vi "Callback.vi"(8 "error in (no error)":errorcluster, 9 "Message Data":variant, 10 "Message":string, 11 "Callback in":refnum<class "Callback.lvclass">) -> (0 "error out":errorcluster)   [LabVIEW 2020, in "Callback.lvclass"]
uses:
  Callback.lvclass
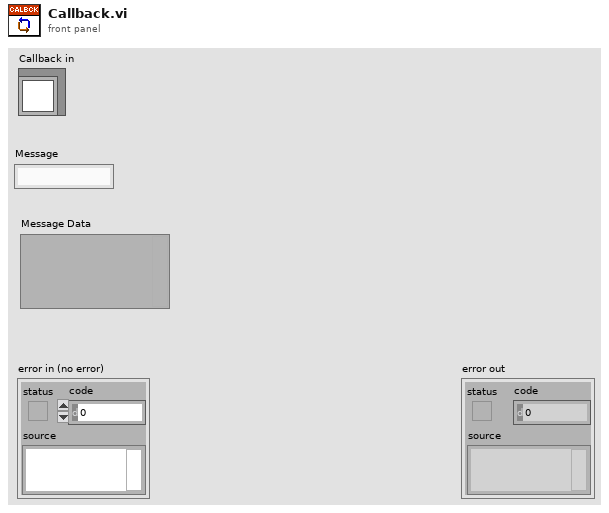
[diagram p1: front panel]
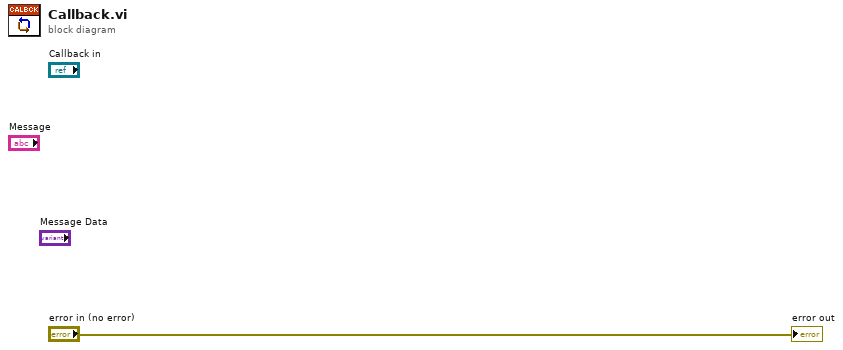
[diagram p0: block diagram]
diagram:
  "error out" <- "error in (no error)"
